vi "VacSafety.vi"(11 "i ref in":refnum<vi>) -> (3 "i ref out":refnum<vi>)   [LabVIEW 2014, in "Panels.lvlib"]
uses:
  Panels.lvlib
panel:
  # "Vacuum Safety"
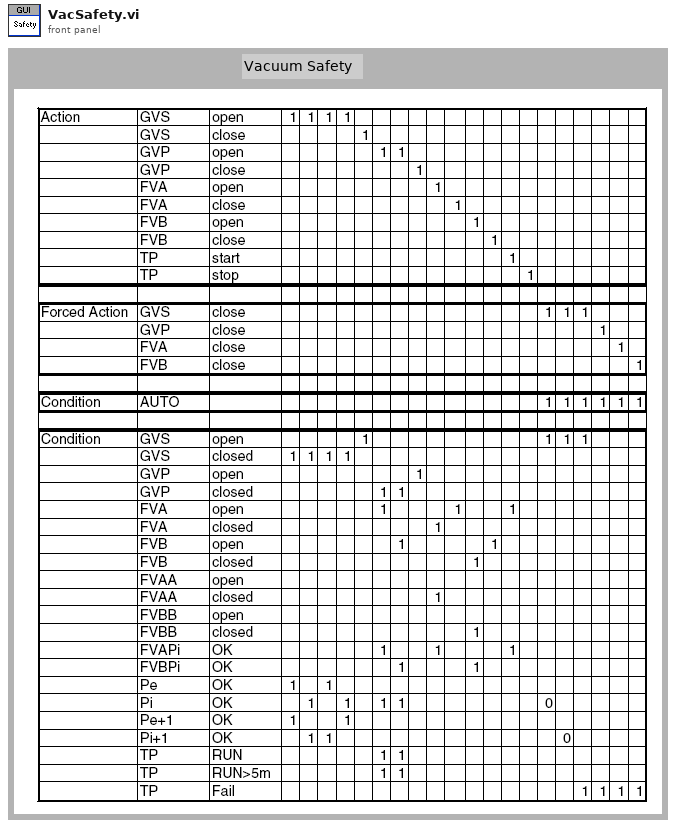
[diagram p1: front panel]
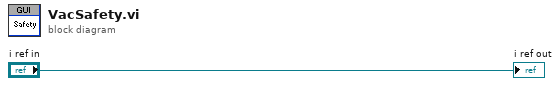
[diagram p0: block diagram]
diagram:
  "i ref out" <- "i ref in"
